vi "_searchDataPlugin.vi"(8 "error in (no error)":errorcluster, 10 "Value":string, 11 "DataPlugin information":T1[](array[typedef])) -> (0 "error out":errorcluster, 2 "Indices":i32[](array[numeric]), 3 "DataPlugin information out":T1[](array[typedef]))   [LabVIEW 2020]
uses:
  <vilib>/Platform/storage/utility/DataPluginSynchronization/_DataPluginInfo.ctl
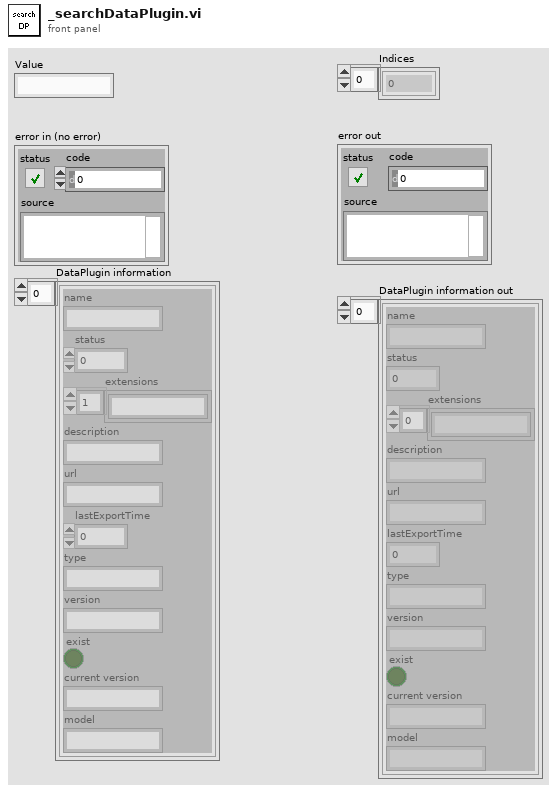
[diagram p1: front panel]
types:
  T1 = typedef "_DataPluginInfo.ctl" = cluster{"name":string, "status":u32, "extensions":string[], "description":string, "url":string, "lastExportTime":i64, "type":string, "version":string, "exist":bool, "current version":string, "model":string}
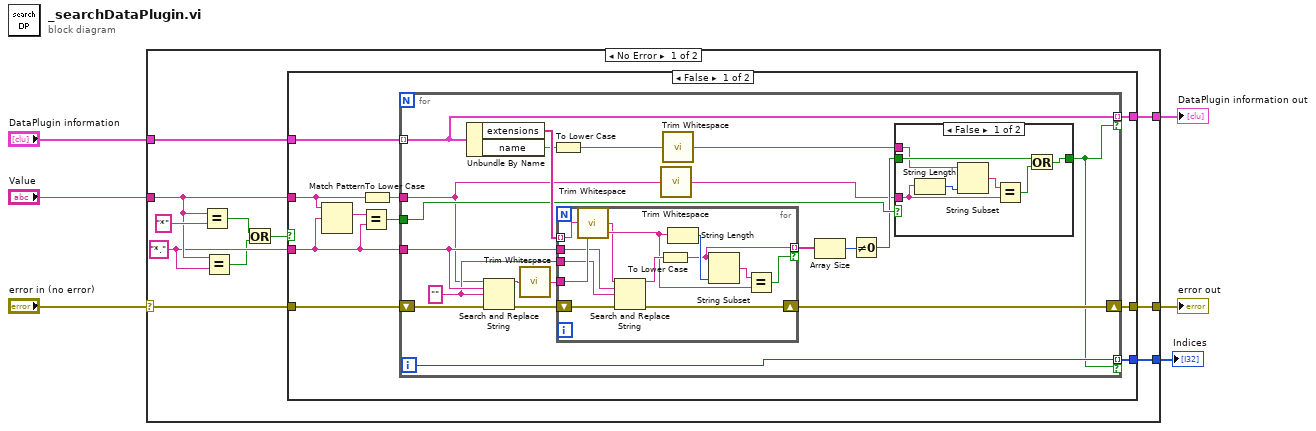
[diagram p0: block diagram]
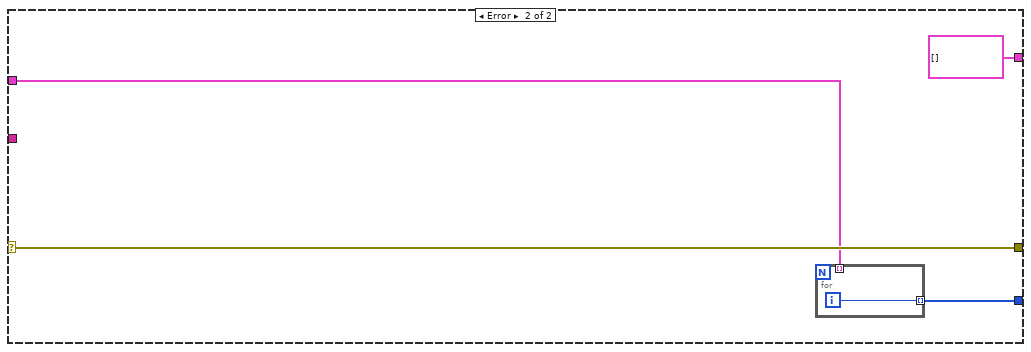
[diagram p4: hidden frame]
diagram:
  n1 = case shown="No Error" "error in (no error)" {
    selector: "error in (no error)" -> [w14 w75]
    tunnel: "Value" -> [w11 _]
    tunnel: "DataPlugin information" -> [w17 w73]
    tunnel: [w15 T1[] []] -> w4
    tunnel: [w16 w75] -> w2
    tunnel: [w13 w72] -> w1
    frame No Error {
      w10 = "*." ("search string")
      n2 = Equal?(x=w11, y="*") -> (x = y?=w9:bool)
      n3 = Equal?(x=w11, y=w10) -> (x = y?=w8:bool)
      n4 = Or(x=w9, y=w8) -> (x .or. y?=w7:bool)
      n5 = case shown="False" w7 {
        tunnel: w17 -> [w25 w69]
        tunnel: [w24 w70] -> w16
        tunnel: [w22 w69] -> w15
        tunnel: w14 -> [w21 w70]
        tunnel: [w20 w68] -> w13
        tunnel: w11 -> [w19 _]
        tunnel: w10 -> [w18 _]
        frame False {
          n6 = Match Pattern(string=w19, regular expression=w18) -> (match substring=w27:string)  [unwired: 1 in, 3 out]
          n7 = Equal?(x=w27, y=w18) -> (x = y?=w23:bool)
          n8 = To Lower Case(string=w19) -> (all lower case string=w26:string)
          n9 = for {
            tunnel: w26 -> [w29]
            tunnel: w25 -> [w46] mode=indexing
            tunnel: [w46] -> w22 mode=indexing if=w34
            shift-right: [w40] -> w24
            shift-left: w21 -> [w42]
            tunnel: w23 -> [w39]
            tunnel: w18 -> [w37]
            tunnel: [w35] -> w20 mode=indexing if=w34
            i -> [w35]
            w36 = "" ("replace string (\"\")")
            n10 = Unbundle By Name(w46) -> ("extensions"=w45:string[], "name"=w43:string)
            n11 = Search and Replace String(input string=w29, search string=w37, replace string=w36, error in=w42) -> (result string=w33:string, error out=w41:errorcluster)  [unwired: 4 in, 2 out]
            n12 = call <vilib>:"Trim Whitespace.vi"("string"=w33) -> ("trimmed string"=w32:string)  [unwired: 1 in]
            n13 = To Lower Case(string=w43) -> (all lower case string=w31:string)
            n14 = for {
              tunnel: w45 -> [w57] mode=indexing
              tunnel: w32 -> [w66]
              tunnel: [w62] -> w44 mode=indexing if=w65
              shift-right: [w60] -> w40
              shift-left: w41 -> [w61]
              tunnel: w37 -> [w59]
              tunnel: w36 -> [w58]
              n15 = call <vilib>:"Trim Whitespace.vi"("string"=w57) -> ("trimmed string"=w56:string)  [unwired: 1 in]
              n16 = Search and Replace String(input string=w56, search string=w59, replace string=w58, error in=w61) -> (result string=w67:string, error out=w60:errorcluster)  [unwired: 4 in, 2 out]
              n17 = To Lower Case(string=w67) -> (all lower case string=w62:string)
              n18 = String Length(string=w66) -> (length=w64:i32)
              n19 = String Subset(string=w62, length (rest)=w64) -> (substring=w63:string)  [unwired: 1 in]
              n20 = Equal?(x=w63, y=w66) -> (x = y?=w65:bool)
            }
            n21 = call <vilib>:"Trim Whitespace.vi"("string"=w29) -> ("trimmed string"=w28:string)  [unwired: 1 in]
            n22 = call <vilib>:"Trim Whitespace.vi"("string"=w31) -> ("trimmed string"=w30:string)  [unwired: 1 in]
            n23 = Array Size(array=w44) -> (size(s)=w47:i32)
            n24 = Not Equal To 0?(x=w47) -> (x != 0?=w38:bool)
            n25 = case shown="False" w39 {
              tunnel: w30 -> [w49 _]
              tunnel: w28 -> [w54 _]
              tunnel: w38 -> [w53 w55]
              tunnel: [w52 w55] -> w34
              frame False {
                n26 = String Length(string=w54) -> (length=w48:i32)
                n27 = String Subset(string=w49, length (rest)=w48) -> (substring=w50:string)  [unwired: 1 in]
                n28 = Equal?(x=w50, y=w54) -> (x = y?=w51:bool)
                n29 = Or(x=w53, y=w51) -> (x .or. y?=w52:bool)
              }
              frame True {
              }
            }
          }
        }
        frame True {
          n30 = for {
            tunnel: [w71] -> w68 mode=indexing
            tunnel: w69 -> [_] mode=indexing
            i -> [w71]
          }
        }
      }
    }
    frame Error {
      n31 = for {
        tunnel: w73 -> [_] mode=indexing
        tunnel: [w76] -> w72 mode=indexing
        i -> [w76]
      }
    }
  }
  "DataPlugin information out" <- w4
  "error out" <- w2
  "Indices" <- w1
